vi "InitMaxonMotor.vi"(0 "PID Loop Period":dbl=0.001 format="%#_13g", 3 "error in (no error)":errorcluster) -> (7 "MotorCtrl":refnum<class "MotorControl.lvclass">, 10 "error out":errorcluster)   [LabVIEW 2014]
uses:
  Classes/MotorControl/MotorControl.lvclass
panel:
  in  "Force Rate (N/min)":cluster{"ForceRateLow":dbl, "ForceRateHigh":dbl}={"ForceRateLow"=300.0, "ForceRateHigh"=10000.0} {"ForceRateHigh" format="%#_13g"; "ForceRateLow" format="%#_13g"}
  in  "TransferRatio":dbl=1.0 format="%#_13g"
  in  "output range":cluster{"output high":dbl, "output low":dbl}={"output high"=0.5, "output low"=-0.3}
  in  "setpoint range":cluster{"setpoint high":dbl, "setpoint low":dbl}={"setpoint high"=60.0, "setpoint low"=3.0}
  in  "PID gains":T1={"proportional gain (Kc)"=0.12, "integral time (Ti, min)"=0.003, "derivative time (Td, min)"=0.001}
  in  "MotorFrictionModel":T2(array[cluster])
  in  "Motor Quantity":i32=7
  in  "MotorConstant(F/V)":dbl[](array[numeric])=[55.0, 55.0, 55.0, 55.0, 55.0, 55.0, 55.0]
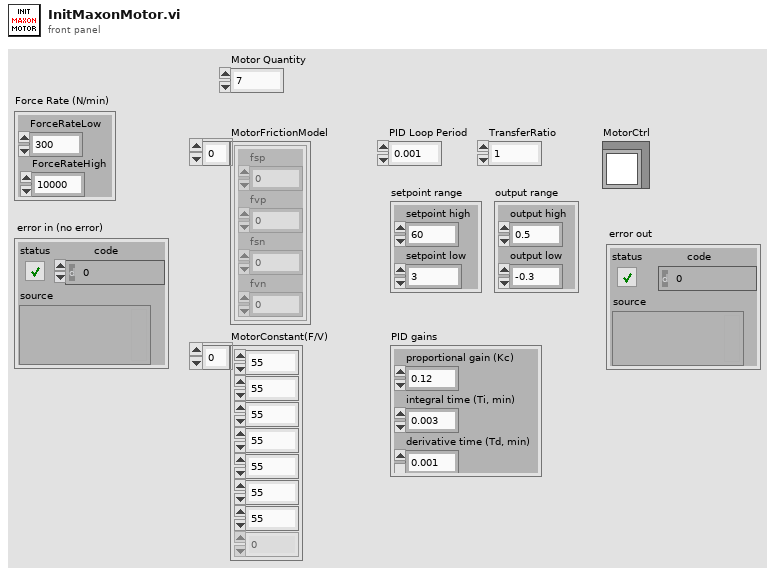
[diagram p1: front panel]
types:
  T1 = cluster{"proportional gain (Kc)":dbl, "integral time (Ti, min)":dbl, "derivative time (Td, min)":dbl}
  T2 = cluster{"fsp":dbl, "fvp":dbl, "fsn":dbl, "fvn":dbl}[]
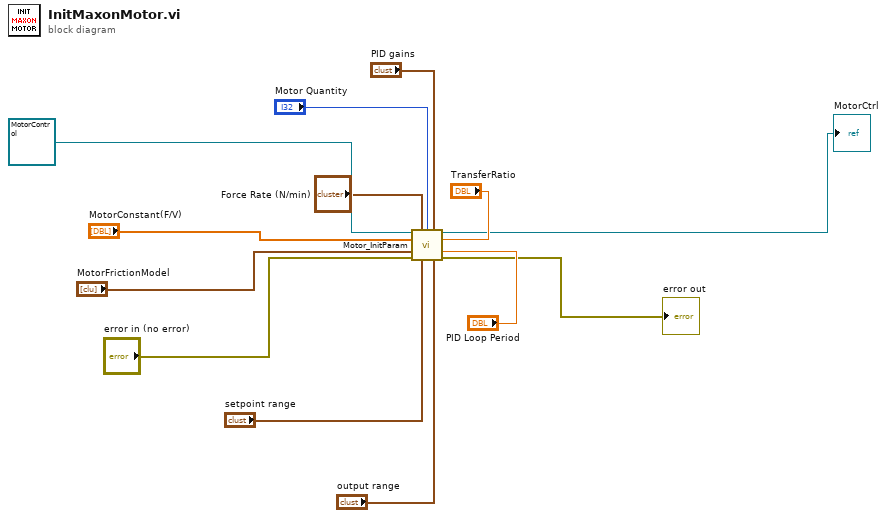
[diagram p0: block diagram]
diagram:
  n1 = call "Motor_InitParam.vi"("Motor Control In"=refnum<class "MotorControl.lvclass"> refnum ("MotorCtrl_In"), "Force Rate (N/min)"="Force Rate (N/min)", "Motor Quantity"="Motor Quantity", "PID gains"="PID gains", "MotorConstant(F/V)"="MotorConstant(F/V)", "TransferRatio"="TransferRatio", "MotorFrictionModel"="MotorFrictionModel", "PID Loop Period"="PID Loop Period", "error in (no error)"="error in (no error)", "output range (N)"="setpoint range", "setpoint range (A)"="output range") -> ("Motor Control Out"=→"MotorCtrl":refnum<class "MotorControl.lvclass">, "error out"=→"error out":errorcluster)  [unwired: 3 in]
